vi "Add Alarm_Alarm and Alarm Folder.vi"(8 "error in (no error)":errorcluster, 9 "Alarm Settings":T1={"Name"="", "Description"="", "Alarm Channel Node Path"="", "UpperLimit"=0.0, "Upper Limit Channel Node Path"="", "LowerLimit"=0.0, "Lower Limit Channel Node Path"="", "Alarm Action Node Path"="", "Mode"=0, "DefaultState"=1, "Priority"=0, "Delay"=0.0, "TripMessage"="", "GroupNumber"=0} {"Priority" items=["Low", "Medium", "High"]; "DefaultState" items=["Disabled", "Enabled"]; "Mode" items=["Normal", "IndicateOnly"]}, 10 "Base Node Path":string, 11 "SysDef Ref":T2) -> (0 "error out":errorcluster, 3 "SysDef Ref Out":T2)   [LabVIEW 2019, in "Simple SysDef API.lvlib"]
uses:
  <userlib>/SimpleSysDef/Simple SysDef API.lvlib
  <userlib>/SimpleSysDef/_SubVIs/System Definition Reference.ctl
  NationalInstruments.VeriStand.SystemDefinitionAPI
  <userlib>/SimpleSysDef/_SubVIs/Add Alarm_Settings.ctl
  <userlib>/SimpleSysDef/_SubVIs/Add Alarm Folder_Settings.ctl
  <userlib>/SimpleSysDef/_SubVIs/Add Alarm Folder.vi
  <userlib>/SimpleSysDef/_SubVIs/Add Alarm.vi
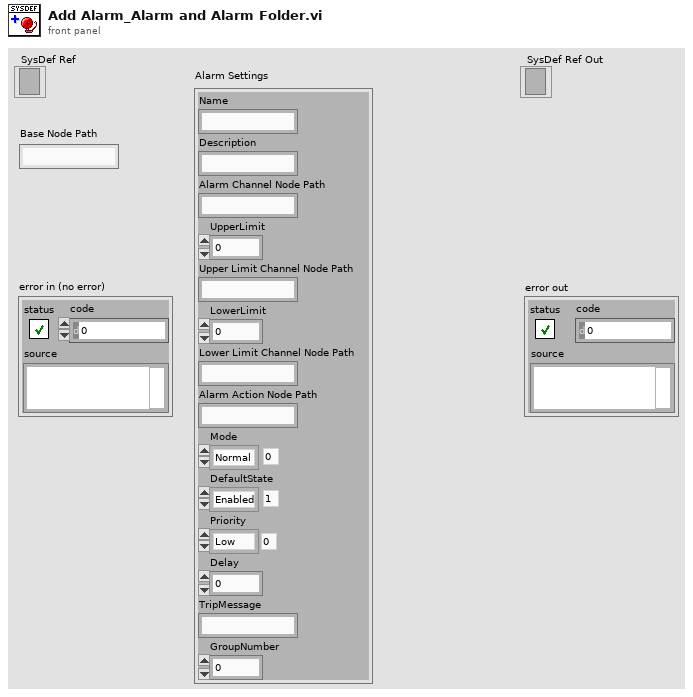
[diagram p1: front panel]
types:
  T1 = typedef "Simple SysDef API.lvlib/Add Alarm_Settings.ctl" = cluster{"Name":string, "Description":string, "Alarm Channel Node Path":string, "UpperLimit":dbl, "Upper Limit Channel Node Path":string, "LowerLimit":dbl, "Lower Limit Channel Node Path":string, "Alarm Action Node Path":string, "Mode":i32, "DefaultState":i32, "Priority":i32, "Delay":dbl, "TripMessage":string, "GroupNumber":u32}
  T2 = typedef "Simple SysDef API.lvlib/System Definition Reference.ctl" = refnum<k24>
  T3 = typedef "Simple SysDef API.lvlib/Add Alarm Folder_Settings.ctl" = cluster{"Name":string, "Description":string}
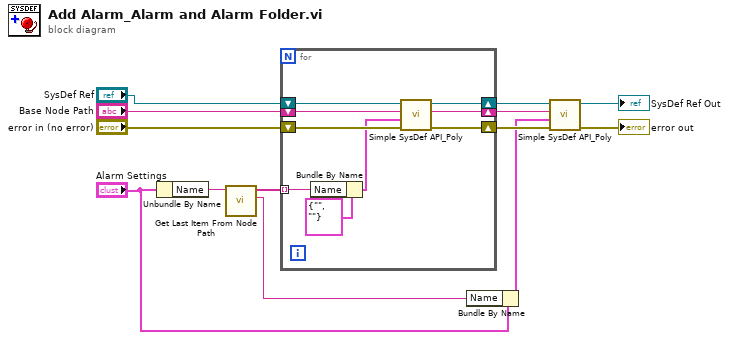
[diagram p0: block diagram]
diagram:
  n1 = Unbundle By Name("Alarm Settings") -> ("Name"=w5:string)
  n2 = call <userlib>:"Get Last Item From Node Path.vi"("Name"=w5) -> ("Last Item"=w2:string, "First Items"=w4:string[])  [unwired: 9 in]
  n3 = for {
    shift-right: [w21] -> w12
    shift-left: "error in (no error)" -> [w18]
    shift-right: [w20] -> w11
    shift-left: "Base Node Path" -> [w17]
    shift-right: [w22] -> w13
    shift-left: "SysDef Ref" -> [w19]
    tunnel: w4 -> [w16] mode=indexing
    n4 = Bundle By Name(cluster=T3 {"Name"="", "Description"=""} ("Alarm Folder"), "Name"=w16) -> (w14:T3)
    n5 = call-poly <userlib>:"Simple SysDef API_Poly.vi"("error in (no error)"=w18, "Alarm Folder"=w14, "Base Node Path"=w17, "SysDef Ref"=w19) -> ("error out"=w21:errorcluster, "New Node Path"=w20:string, "SysDef Ref Out"=w22:T2)  [unwired: 5 in]
  }
  n6 = Bundle By Name(cluster="Alarm Settings", "Name"=w2) -> (w1:T1)
  n7 = call-poly <userlib>:"Simple SysDef API_Poly.vi"("error in (no error)"=w12, "Alarm Settings"=w1, "Base Node Path"=w11, "SysDef Ref"=w13) -> ("error out"=→"error out":errorcluster, "SysDef Ref Out"=→"SysDef Ref Out":T2)  [unwired: 5 in, 1 out]
